vi "MultiColumnListbox_Resize_Absolute.vi"(6 "Flex Column Index":i32, 7 "Parent VI Reference":refnum<vi>, 8 "error in (no error)":errorcluster, 9 "Fit to pane?":bool, 10 "Column Widths [px]":u32[](array[numeric]), 11 "MCLB in":refnum<vi>) -> (0 "error out":errorcluster)   [LabVIEW 2014, in "hse-ui.lvlib"]
doc: "Resizes the columns of a MCLB according to the widths given in <b>Column Widths [px]</b>.The column with the index in <b>Flex Column Index</b> uses the remaining space. If <b>Parent VI Reference</b> is supplied, panel updates are deferred.\n\n____\nHAMPEL SOFTWARE ENGINEERING v0.7.0 (2018-07-16 18:12)"
uses:
  hse-ui.lvlib
  <vilib>/Utility/miscctls.llb/LVRowAndColumnTypeDef.ctl
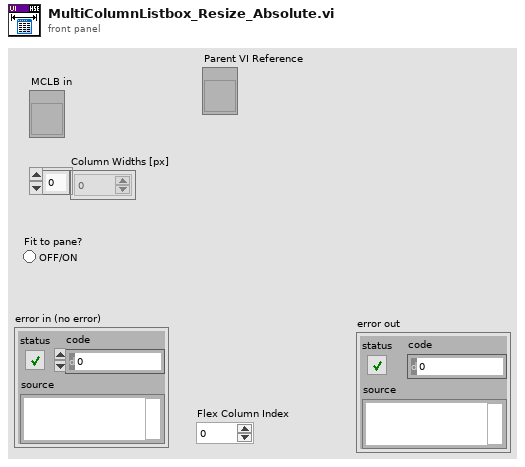
[diagram p1: front panel]
types:
  T1 = typedef "LVRowAndColumnTypeDef.ctl" = cluster{"Row":i32, "Column":i32}
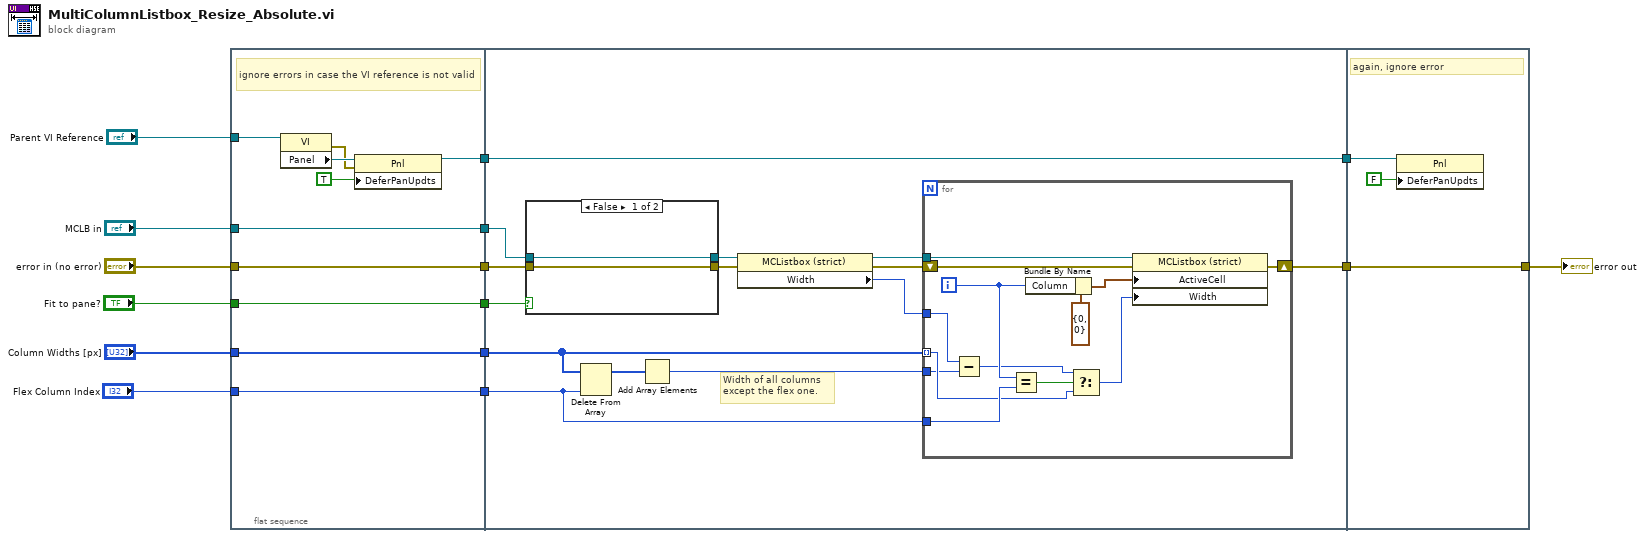
[diagram p0: block diagram]
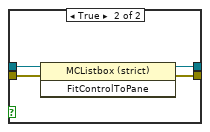
[diagram p2: hidden frame]
diagram:
  n1 = flat-sequence {
    tunnel: "Fit to pane?" -> [w22]
    tunnel: "error in (no error)" -> [w23]
    tunnel: "Column Widths [px]" -> [w24]
    tunnel: "MCLB in" -> [w25]
    tunnel: [w25] -> w9
    tunnel: [w24] -> w8
    tunnel: [w23] -> w7
    tunnel: [w22] -> w6
    tunnel: "Parent VI Reference" -> [w18]
    tunnel: [w17] -> w4
    tunnel: [w16] -> w2
    tunnel: "Flex Column Index" -> [w16]
    tunnel: [w33] -> w10
    tunnel: w9 -> [w39]
    tunnel: w8 -> [w29]
    tunnel: w7 -> [w35]
    tunnel: w6 -> [w32]
    tunnel: [w31] -> w5
    tunnel: w4 -> [w31]
    tunnel: w2 -> [w26]
    tunnel: [w61] -> w12
    tunnel: w10 -> [w61]
    tunnel: w5 -> [w59]
    frame #0 {
      # "ignore errors in case the VI reference is not valid"
      n2 = property class="VI"(reference=w18) -> (error out=w20:errorcluster, "Panel"=w21:refnum<vi>)  [unwired: 1 in, 1 out]
      n3 = property class="Pnl"(reference=w21, error in=w20, "DeferPanUpdts"=TRUE ("Defer Panel Updates")) -> (reference out=w17:refnum<vi>)  [unwired: 1 out]
    }
    frame #1 {
      # "Width of all columns\nexcept the flex one."
      n4 = case shown="False" w32 {
        tunnel: w39 -> [w41 w45]
        tunnel: [w40 w44] -> w37
        tunnel: [w41 w43] -> w36
        tunnel: w35 -> [w40 w42]
        frame False {
        }
        frame True {
          n5 = invoke class="MCListbox (strict)" method="FitControlToPane"(reference=w45, error in=w42) -> (reference out=w43:refnum<vi>, error out=w44:errorcluster)  [unwired: 1 in, 1 out]
        }
      }
      n6 = Delete From Array(array=w29, index=w26) -> (array with subset deleted=w28:u32[])  [unwired: 1 in, 1 out]
      n7 = Add Array Elements(numeric array=w28) -> (sum=w27:u32)
      n8 = property on="Property Node" class="MCListbox (strict)"(reference=w36, error in=w37) -> (reference out=w38:refnum<vi>, error out=w34:errorcluster, "Width"=w30:u32)
      n9 = for {
        tunnel: w29 -> [w50] mode=indexing
        tunnel: w38 -> [w56]
        shift-right: [w54] -> w33
        shift-left: w34 -> [w55]
        tunnel: w30 -> [w47]
        tunnel: w27 -> [w48]
        tunnel: w26 -> [w53]
        i -> [w52]
        n10 = Subtract(x=w47, y=w48) -> (x-y=w46:u32)
        n11 = Equal?(x=w52, y=w53) -> (x = y?=w51:bool)
        n12 = Bundle By Name(cluster=T1 {"Row"=0, "Column"=0} ("Active Cell:Active Cell"), "Column"=w52) -> (w57:T1)
        n13 = Select(t=w46, s=w51, f=w50) -> (s? t:f=w49:u32)
        n14 = property on="Property Node" class="MCListbox (strict)"(reference=w56, error in=w55, "ActiveCell"=w57, "Width"=w49) -> (error out=w54:errorcluster)  [unwired: 1 out]
      }
    }
    frame #2 {
      # "again, ignore error"
      n15 = property class="Pnl"(reference=w59, "DeferPanUpdts"=FALSE ("Defer Panel Updates")) -> ()  [unwired: 1 in, 2 out]
    }
  }
  "error out" <- w12
